vi "image_buffer_length.vi"(7 "LabVIEW Web Service Request":refnum<class "Web Request.lvclass">) -> (2 "ImageBufferLength":i32)   [LabVIEW 2017]
uses:
  <vilib>/wsapi/Web Request.lvclass
  SystemController/SystemController.lvclass
panel:
  # "Use the Web Service Request input terminal to call the VIs on the Web Services palette. Do not remove it from the connector pane unless you don't need access to the palette."
  # "Each additional control wired to the connector pane will be available as an input in the URL. To include an indicator in terminal-mode output (the default setting), it must also be wired to the connector pane."
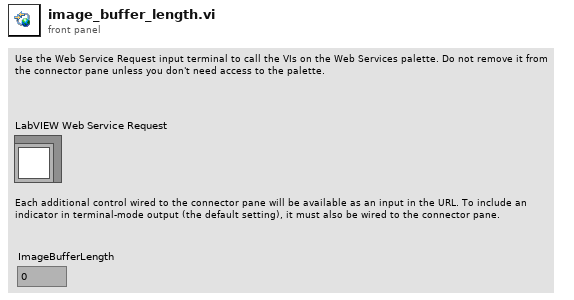
[diagram p1: front panel]
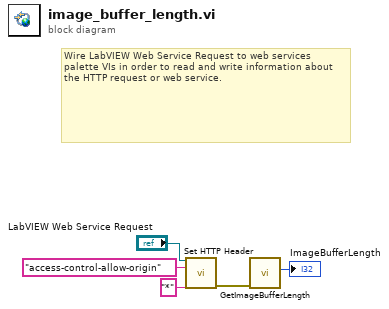
[diagram p0: block diagram]
diagram:
  # "Wire LabVIEW Web Service Request to web services palette VIs in order to read and write information about the HTTP request or web service."
  n1 = call <vilib>:"Set HTTP Header.vi"("LabVIEW Web Service Request"="LabVIEW Web Service Request", "header"="access-control-allow-origin", "header value"="*") -> ("error out"=w1:errorcluster)  [unwired: 11 in, 1 out]
  n2 = call "GetImageBufferLength.vi"("error in (no error)"=w1) -> ("Image Buffer Length"=→"ImageBufferLength":i32)  [unwired: 9 in, 1 out]
